vi "Min Max and Ave.vi"(0 "Data In":sgl[](array[numeric]) format="%.2f") -> (1 "Ave. Pressure Input":sgl format="%.2f", 2 "# Pts, Min, Max, Ave.":sgl[](array[numeric]) format="%.2f")   [LabVIEW 2013]
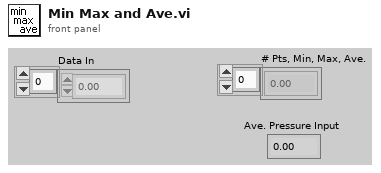
[diagram p1: front panel]
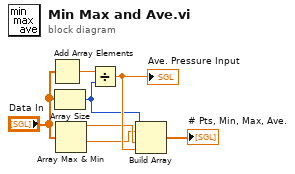
[diagram p0: block diagram]
diagram:
  n1 = Add Array Elements(numeric array="Data In") -> (sum=w5:sgl)
  n2 = Array Size(array="Data In") -> (size(s)=w1:i32)
  n3 = Array Max & Min(array="Data In") -> (max value=w4:sgl, min value=w3:sgl)  [unwired: 2 out]
  n4 = Divide(x=w5, y=w1) -> (x/y=w7:sgl)
  "Ave. Pressure Input" <- w7
  n5 = Build Array(w1, w3, w4, w7) -> (→"# Pts, Min, Max, Ave.":sgl[])
